vi "Launcher-state.vi"() -> ()   [LabVIEW 2014]
panel:
  in  "Action?":bool
  in  "Launcher State":T1(ring)
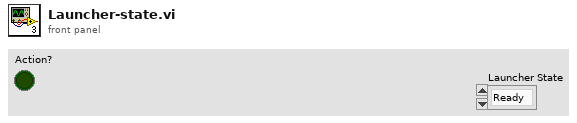
[diagram p1: front panel]
types:
  T1 = enum16{"Ready", "Countdown", "Fire", "Engine Stop", "Abort"}
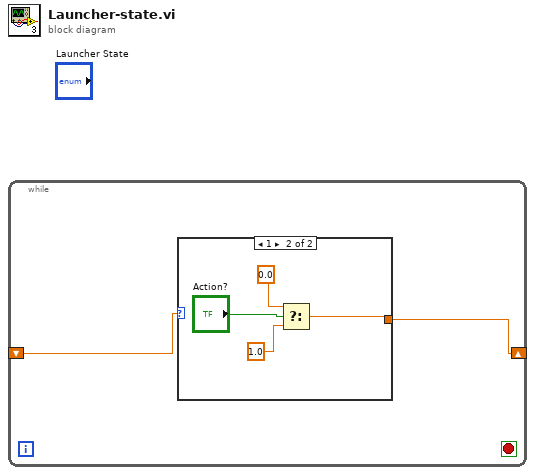
[diagram p0: block diagram]
diagram:
  n1 = while {
    shift-right: [w2] -> _
    shift-left: _ -> [w1]
    stop <- _ stop-if-true
    n2 = case shown="1" w1 {
      tunnel: [_ w3] -> w2
      frame 0, Default {
      }
      frame 1 {
        n3 = Select(t=0.0, s="Action?", f=1.0) -> (s? t:f=w3:dbl)
      }
    }
  }
